vi "UI ADLINK Motion Card.vi"(8 "error in (no error)":errorcluster, 11 "Module Name":string="Axis") -> (0 "error out":errorcluster)   [LabVIEW 2019, in "ADLINK Motion Card.lvlib"]
uses:
  ADLINK Motion Card.lvlib
  User Event/Controls/UE Abort Action.ctl
  <vilib>/Utility/miscctls.llb/LVPointTypeDef.ctl
  Queues/Queues.lvlib
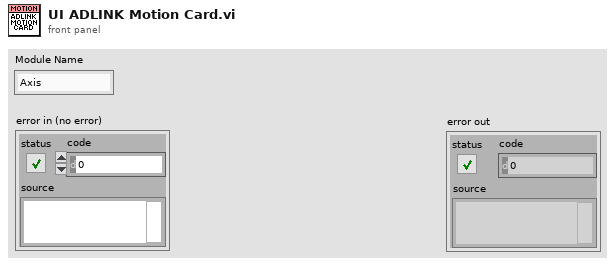
[diagram p1: front panel]
types:
  T1 = typedef "UE Abort Action.ctl" = enum16{"Create", "Get", "Destroy"}
  T2 = typedef "LVPointTypeDef.ctl" = cluster{"Horizontal":i16, "Vertical":i16}
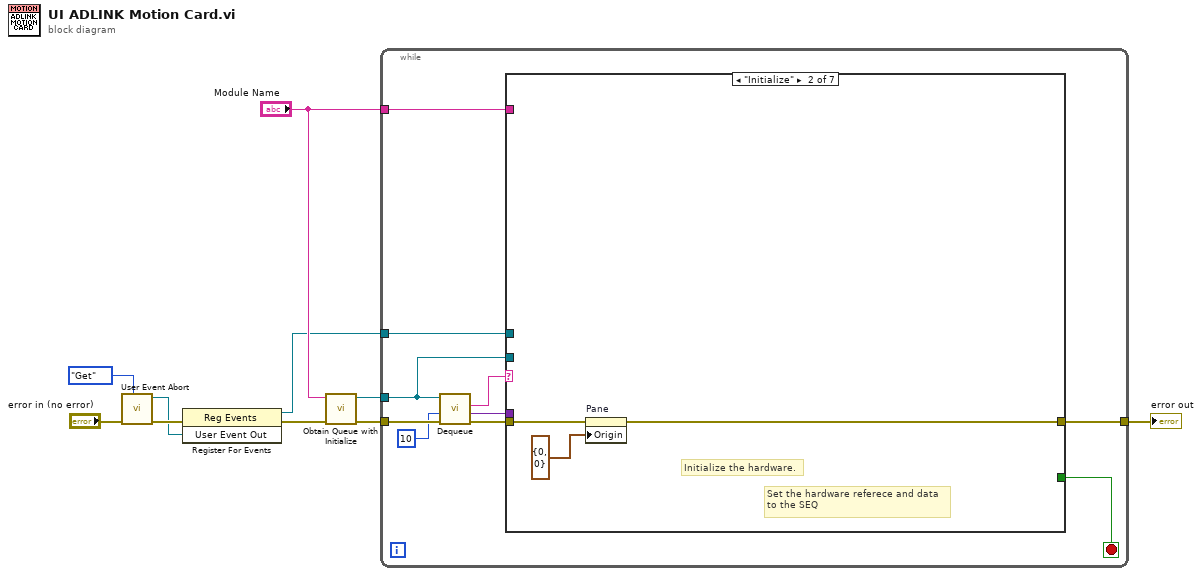
[diagram p0: block diagram]
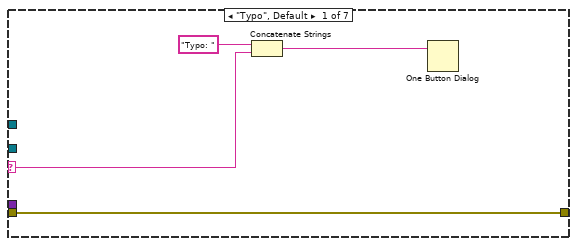
[diagram p2: hidden frame]
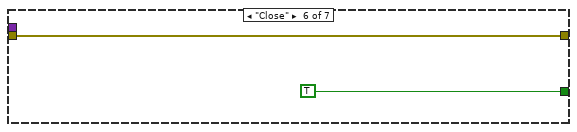
[diagram p6: hidden frame]
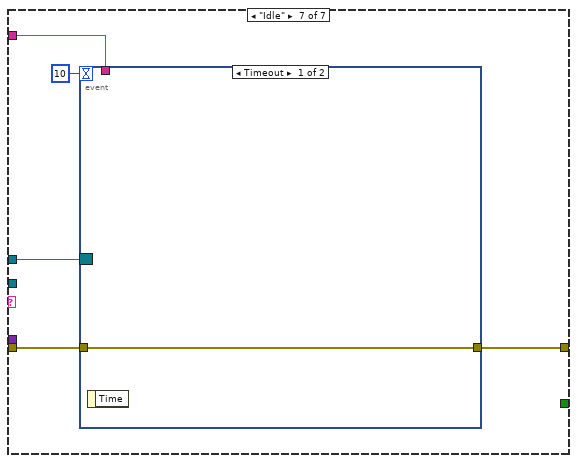
[diagram p7: hidden frame]
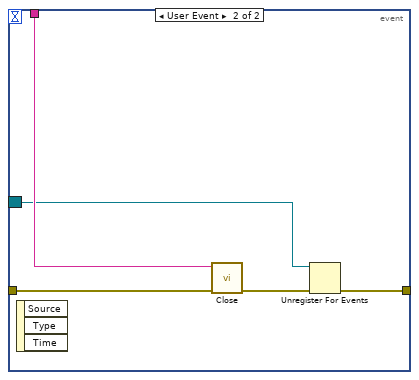
[diagram p8: hidden frame]
diagram:
  n1 = call "User Event Abort.vi"("Action"=UE_Abort_Action."Get", "Error In"="error in (no error)") -> ("Error Out"=w5:errorcluster, "User Event Out"=w4:refnum<user-event>)  [unwired: 8 in]
  n2 = register-events(error in=w5, w4) -> (reference out=w1:refnum<event-registration>, error out=w2:errorcluster)  [unwired: 1 in]
  n3 = call "Obtain Queue with Initialize.vi"("Error In"=w2, "Queue Name"="Module Name") -> ("Error Out"=w9:errorcluster, "Queue out"=w10:refnum<queue>)  [unwired: 8 in]
  n4 = while {
    tunnel: w9 -> [w20]
    tunnel: w10 -> [w13]
    tunnel: [w15] -> w8
    tunnel: "Module Name" -> [w14]
    tunnel: w1 -> [w12]
    stop <- w11 stop-if-true
    n5 = call "Dequeue.vi"("Error In"=w20, "timeout in ms (-1)"=10, "Queue in"=w13) -> ("Error Out"=w18:errorcluster, "Data"=w16:variant, "State"=w17:string)  [unwired: 5 in, 1 out]
    n6 = case shown="\"Initialize\"" w17 {
      selector: w17 -> [w22 _ _ _ _ _ _]
      tunnel: w18 -> [w21 w26 w28 w29 w30 w31 w36]
      tunnel: w16 -> [_ _ _ _ _ _ _]
      tunnel: [w21 w25 w28 w29 w30 w31 w35] -> w15
      tunnel: w14 -> [_ _ _ _ _ _ w33]
      tunnel: w13 -> [_ _ _ _ _ _ _]
      tunnel: w12 -> [_ _ _ _ _ _ w34]
      tunnel: [_ _ _ _ _ TRUE ("force destroy? (F)") _] -> w11
      frame "Typo", Default {
        n7 = Concatenate Strings("Typo: " ("string"), w22) -> (w24:string)
        n8 = One Button Dialog(message=w24) -> ()  [unwired: 1 in, 1 out]
      }
      frame "Initialize" {
        # "Set the hardware referece and data\nto the SEQ"
        # "Initialize the hardware."
        n9 = property on="Pane" class="Pane"(error in=w26, "Origin"=T2 {"Horizontal"=0, "Vertical"=0}) -> (error out=w25:errorcluster)  [unwired: 1 in, 1 out]
      }
      frame "Set" {
        # "Write the new setting\nto the hardware."
      }
      frame "Move" {
        # "Send the command to hardware.\nAsk the motor move to the target position."
      }
      frame "Check" {
        # "Read the Hardware Position"
      }
      frame "Close" {
      }
      frame "Idle" {
        n10 = event shown="[0] Timeout" {
          selector: w34 -> [_ w40]
          dyn-events: _ -> [_ _]
          timeout: 10 -> [_ _]
          tunnel: w36 -> [w38 w43]
          tunnel: [w38 w39] -> w35
          tunnel: w33 -> [_ w42]
          event Timeout {
            n11 = event-data() -> ()  [unwired: 1 in, 1 out]
          }
          event User Event {
            n12 = event-data() -> ()  [unwired: 1 in, 3 out]
            n13 = call "Close.vi"("error in (no error)"=w43, "Queue Name"=w42) -> ("error out"=w41:errorcluster)  [unwired: 9 in]
            n14 = Unregister For Events(event registration refnum=w40, error in=w41) -> (error out=w39:errorcluster)
          }
        }
      }
    }
  }
  "error out" <- w8
